vi "home_az.vi"(10 "angle":dbl, 11 "output cluster in":T1) -> (3 "output cluster out":T1)   [LabVIEW 2015, in "PolyVIEW.lvclass"]
uses:
  PolyVIEW.lvclass
  Memory.ctl
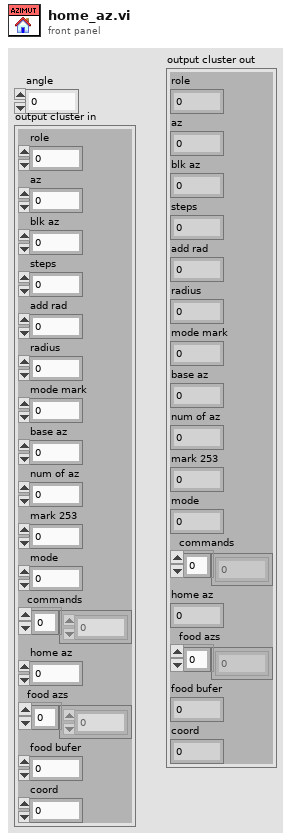
[diagram p1: front panel]
types:
  T1 = typedef "PolyVIEW.lvclass/Memory.ctl" = cluster{"role":i32, "az":i32, "blk az":i32, "steps":dbl, "add rad":i32, "radius":dbl, "mode mark":u32, "base az":dbl, "num of az":u32, "mark 253":u32, "mode":u32, "commands":i32[], "home az":dbl, "food azs":dbl[], "food bufer":dbl, "coord":cdb}
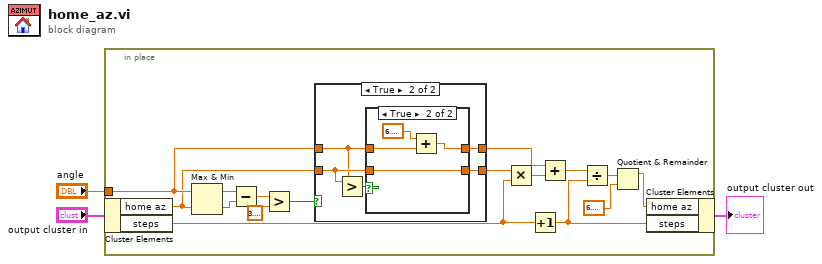
[diagram p0: block diagram]
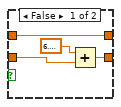
[diagram p3: hidden frame]
diagram:
  n1 = in-place {
    in-place-border: "angle" -> [w8]
    n2 = in-place-cluster #1("output cluster in") -> ("home az"=w7:dbl, "steps"=w10:dbl)
    n3 = Max & Min(x=w8, y=w7) -> (max(x,y)=w17:dbl, min(x,y)=w16:dbl)
    n4 = Subtract(x=w17, y=w16) -> (x-y=w15:dbl)
    n5 = Greater?(x=w15, y=3.141592653589793) -> (0:w13:bool)
    n6 = case shown="True" w13 {
      tunnel: w7 -> [w21 w25]
      tunnel: w8 -> [w20 w24]
      tunnel: [w21 w23] -> w12
      tunnel: [w20 w22] -> w11
      frame False {
      }
      frame True {
        n7 = Greater?(x=w25, y=w24) -> (0:w26:bool)
        n8 = case shown="True" w26 {
          tunnel: w25 -> [w29 w34]
          tunnel: w24 -> [w27 w33]
          tunnel: [w28 w34] -> w23
          tunnel: [w27 w31] -> w22
          frame False {
            n9 = Add(x=6.283185307179586, y=w29) -> (x+y=w28:dbl)
          }
          frame True {
            n10 = Add(x=6.283185307179586, y=w33) -> (x+y=w31:dbl)
          }
        }
      }
    }
    n11 = Multiply(x=w12, y=w10) -> (x*y=w19:dbl)
    n12 = Increment(x=w10) -> (x+1=w9:dbl)
    n13 = Add(x=w11, y=w19) -> (x+y=w18:dbl)
    n14 = Divide(x=w18, y=w9) -> (x/y=w6:dbl)
    n15 = Quotient & Remainder(x=w6, y=6.283185307179586) -> (x-y*floor(x/y)=w4:dbl)  [unwired: 1 out]
    n16 = in-place-cluster #1("home az"=w4, "steps"=w9) -> (→"output cluster out":T1)
  }
